vi "MovePostion.vi"(8 "error in (no error)":errorcluster, 10 "position":dbl) -> (0 "error out":errorcluster, 1 "MoveDisance":string)   [LabVIEW 2017]
uses:
  C:/x682_Camera_Program/X682 Camera Calibration Tester Program/Thorlabs.MotionControl.Controls.dll
  Thorlabs.MotionControl.Controls.dll
  C:/x682_Camera_Program/X682 Camera Calibration Tester Program/Thorlabs.MotionControl.IntegratedStepperMotorsCLI.dll
  Thorlabs.MotionControl.IntegratedStepperMotorsCLI.dll
panel:
  in  "LongTravelStageControl":refnum<k24>(container)
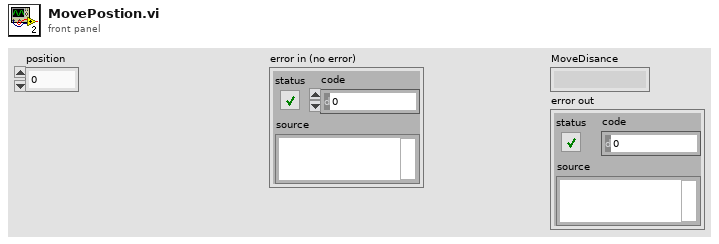
[diagram p1: front panel]
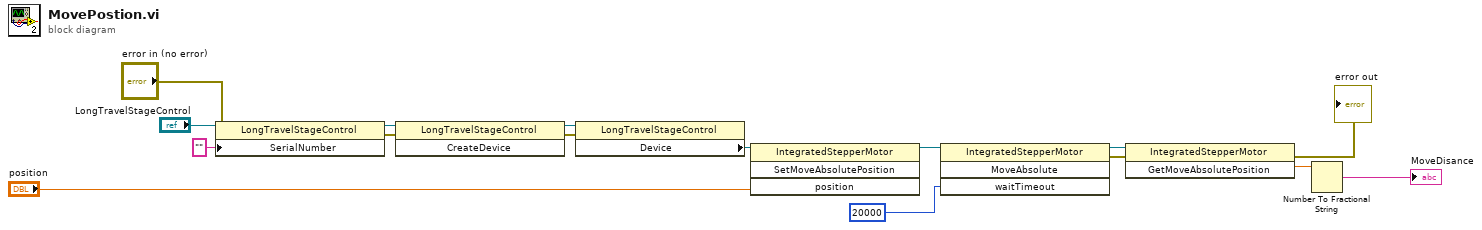
[diagram p0: block diagram]
diagram:
  n1 = property class="LongTravelStageControl"(reference="LongTravelStageControl", error in="error in (no error)", "SerialNumber"="") -> (reference out=w14:refnum<k24>, error out=w12:errorcluster)
  n2 = invoke class="LongTravelStageControl" method="CreateDevice"(reference=w14, error in=w12) -> (reference out=w13:refnum<k24>, error out=w11:errorcluster)  [unwired: 1 in, 1 out]
  n3 = property class="LongTravelStageControl"(reference=w13, error in=w11) -> ("Device"=w15:refnum<k24>)  [unwired: 2 out]
  n4 = invoke class="IntegratedStepperMotor" method="SetMoveAbsolutePosition"(reference=w15, "position"="position") -> (reference out=w16:refnum<k24>)  [unwired: 2 in, 3 out]
  n5 = invoke class="IntegratedStepperMotor" method="MoveAbsolute"(reference=w16, "waitTimeout"=20000) -> (reference out=w5:refnum<k24>, error out=w7:errorcluster)  [unwired: 2 in, 2 out]
  n6 = invoke class="IntegratedStepperMotor" method="GetMoveAbsolutePosition"(reference=w5, error in=w7) -> (error out=→"error out":errorcluster, "GetMoveAbsolutePosition"=w6:dbl)  [unwired: 1 in, 1 out]
  n7 = Number To Fractional String(number=w6) -> (F-format string=→"MoveDisance":string)  [unwired: 3 in]
